vi "Deadzone.vi"(10 "Deadzone":dbl, 11 "Value":dbl) -> (2 "Inside Deadzone?":bool, 3 "Numeric":dbl)   [LabVIEW 2018]
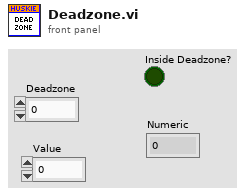
[diagram p1: front panel]
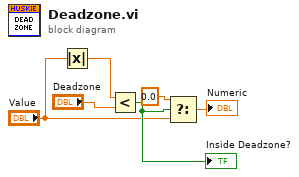
[diagram p0: block diagram]
diagram:
  n1 = Absolute Value(x="Value") -> (abs(x)=w4:dbl)
  n2 = Less?(x=w4, y="Deadzone") -> (x < y?=w5:bool)
  "Inside Deadzone?" <- w5
  n3 = Select(t=0.0, s=w5, f="Value") -> (s? t:f=→"Numeric":dbl)
